vi "Autoarrange Plots.vi"(0 "Data in":T7, 5 "Display State":T3, 9 "panel":refnum<vi>) -> (4 "Data out":T2(array[cluster]), 15 "error out":errorcluster)   [LabVIEW 2015, in "Interactive Graph.xctl"]
uses:
  Interactive Graph.xctl
  Data.vi
  EPhys/LV Source/Work Panel VIs/Typedefs/EPhysWork-Label Position.ctl
  State.vi
  Persistent.ctl
  Plot.ctl
  Events.ctl
  Selection.ctl
  XRange.ctl
  YScale.ctl
  Cursor.ctl
  <vilib>/Analysis/baseanly.llb/Mean (DBL).vi
  <vilib>/Analysis/NI_AALBase.lvlib
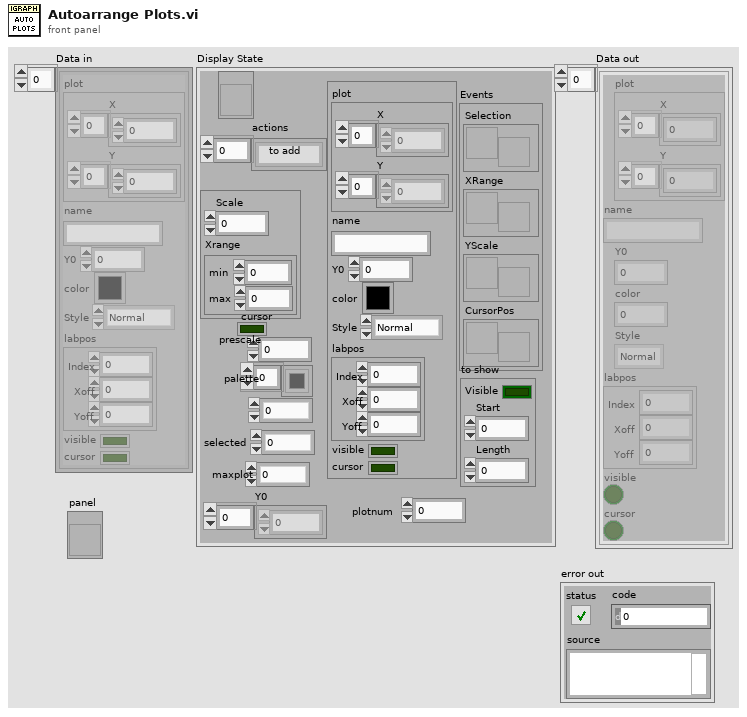
[diagram p1: front panel]
types:
  T1 = typedef "EPhysWork-Label Position.ctl" = cluster{"Index":i32, "Xoff":dbl, "Yoff":dbl}
  T2 = cluster{"plot":cluster{"X":dbl[], "Y":dbl[]}, "name":string, "Y0":dbl, "color":u32, "Style":enum16{"Normal", "Highlight", "Shadow"}, "labpos":T1, "visible":bool, "cursor":bool}[]
  T3 = typedef "Interactive Graph.xctl/State.vi" = cluster{"ref":refnum<vi>, "actions":string[], "Persist":T4, "cursor":bool, "prescale":dbl, "palette":u32[], "colIndex":i32, "to add":T5, "Events":T6, "selected":i32, "to show":cluster{"Visible":bool, "Start":i32, "Length":i32}, "maxplot":i32, "Y0":dbl[], "plotnum":i32}
  T4 = typedef "Interactive Graph.xctl/Persistent.ctl" = cluster{"Scale":dbl, "Xrange":cluster{"min":dbl, "max":dbl}}
  T5 = typedef "Interactive Graph.xctl/Plot.ctl" = cluster{"plot":cluster{"X":dbl[], "Y":dbl[]}, "name":string, "Y0":dbl, "color":u32, "Style":enum16{"Normal", "Highlight", "Shadow"}, "labpos":T1, "visible":bool, "cursor":bool}
  T6 = typedef "Interactive Graph.xctl/Events.ctl" = cluster{"Selection":refnum<user-event>, "XRange":refnum<user-event>, "YScale":refnum<user-event>, "CursorPos":refnum<user-event>}
  T7 = typedef "Interactive Graph.xctl/Data.vi" = cluster{"plot":cluster{"X":dbl[], "Y":dbl[]}, "name":string, "Y0":dbl, "color":u32, "Style":enum16{"Normal", "Highlight", "Shadow"}, "labpos":T1, "visible":bool, "cursor":bool}[]
  T8 = cluster{"plot":cluster{"X":dbl[], "Y":dbl[]}, "name":string, "Y0":dbl, "color":u32, "Style":enum16{"Normal", "Highlight", "Shadow"}, "labpos":T1, "visible":bool, "cursor":bool}
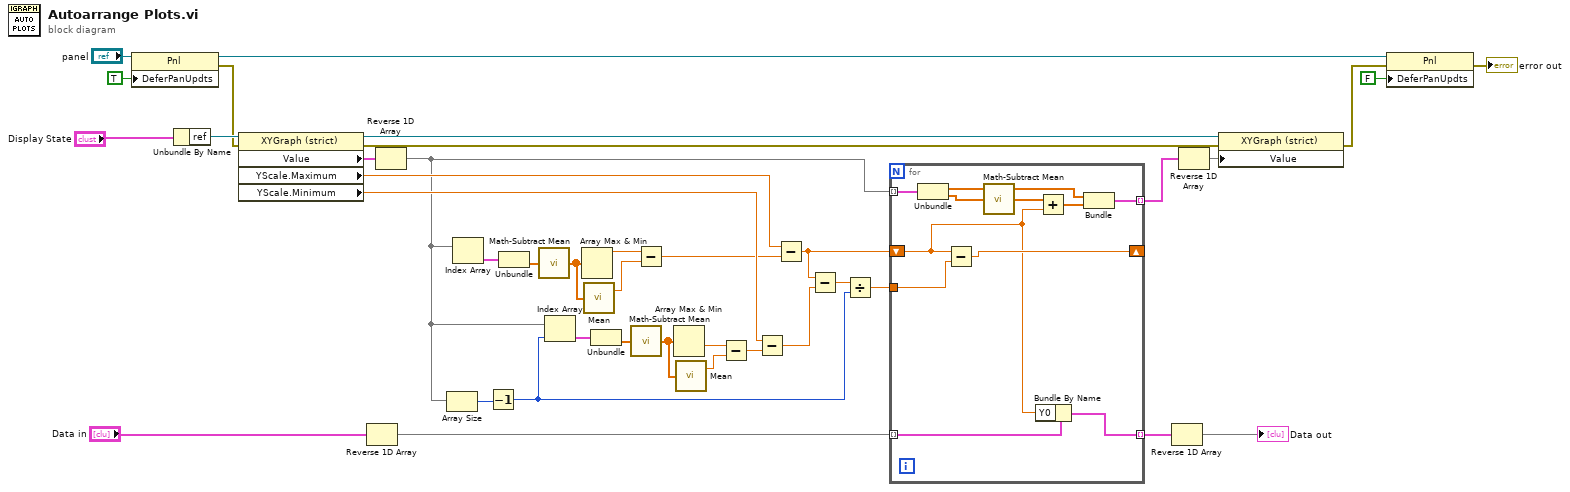
[diagram p0: block diagram]
diagram:
  n1 = property class="Pnl"(reference="panel", "DeferPanUpdts"=TRUE ("Defer Panel Updates")) -> (reference out=w36:refnum<vi>, error out=w7:errorcluster)  [unwired: 1 in]
  n2 = Unbundle By Name("Display State") -> ("ref"=w9:refnum<vi>)
  n3 = property class="XYGraph (strict)"(reference=w9, error in=w7) -> (reference out=w27:refnum<vi>, error out=w28:errorcluster, "Value"=w29:cluster{dbl[], dbl[]}[], "YScale.Maximum"=w30:dbl, "YScale.Minimum"=w31:dbl)
  n4 = Reverse 1D Array(array="Data in") -> (reversed array=w3:T7)
  n5 = Reverse 1D Array(array=w29) -> (reversed array=w4:cluster{dbl[], dbl[]}[])
  n6 = Array Size(array=w4) -> (size(s)=w26:i32)
  n7 = Index Array(array=w4) -> (element=w24:cluster{dbl[], dbl[]})  [unwired: 1 in]
  n8 = Decrement(x=w26) -> (x-1=w32:i32)
  n9 = Unbundle(w24) -> (w23:dbl[])  [unwired: 1 out]
  n10 = call "Math-Subtract Mean.vi"("Y"=w23) -> ("Y - mean(Y)"=w22:dbl[])  [unwired: 4 in]
  n11 = Index Array(array=w4, index=w32) -> (element=w19:cluster{dbl[], dbl[]})
  n12 = Array Max & Min(array=w22) -> (max value=w21:dbl)  [unwired: 3 out]
  n13 = call-poly <vilib>:"Mean.vi"("X"=w22) -> ("mean"=w20:dbl)  [unwired: 1 out]
  n14 = Unbundle(w19) -> (w18:dbl[])  [unwired: 1 out]
  n15 = call "Math-Subtract Mean.vi"("Y"=w18) -> ("Y - mean(Y)"=w17:dbl[])  [unwired: 4 in]
  n16 = Subtract(x=w21, y=w20) -> (x-y=w25:dbl)
  n17 = Array Max & Min(array=w17) -> (min value=w15:dbl)  [unwired: 3 out]
  n18 = call-poly <vilib>:"Mean.vi"("X"=w17) -> ("mean"=w16:dbl)  [unwired: 1 out]
  n19 = Subtract(x=w15, y=w16) -> (x-y=w14:dbl)
  n20 = Subtract(x=w31, y=w14) -> (x-y=w12:dbl)
  n21 = Subtract(x=w30, y=w25) -> (x-y=w13:dbl)
  n22 = Subtract(x=w13, y=w12) -> (x-y=w11:dbl)
  n23 = Divide(x=w11, y=w32) -> (x/y=w10:dbl)
  n24 = for {
    shift-right: [w50] -> _
    shift-left: w13 -> [w41]
    tunnel: w10 -> [w49]
    tunnel: w4 -> [w44] mode=indexing
    tunnel: [w43] -> w33 mode=indexing
    tunnel: w3 -> [w42] mode=indexing
    tunnel: [w40] -> w5 mode=indexing
    n25 = Unbundle(w44) -> (w46:dbl[], w48:dbl[])
    n26 = Subtract(x=w41, y=w49) -> (x-y=w50:dbl)
    n27 = call "Math-Subtract Mean.vi"("Y"=w48) -> ("Y - mean(Y)"=w45:dbl[])  [unwired: 4 in]
    n28 = Bundle By Name(cluster=w42, "Y0"=w41) -> (w40:T8)
    n29 = Add(x=w45, y=w41) -> (x+y=w47:dbl[])
    n30 = Bundle(w46, w47) -> (w43:cluster{dbl[], dbl[]})  [unwired: 1 in]
  }
  n31 = Reverse 1D Array(array=w5) -> (reversed array=→"Data out":T2)
  n32 = Reverse 1D Array(array=w33) -> (reversed array=w1:cluster{dbl[], dbl[]}[])
  n33 = property class="XYGraph (strict)"(reference=w27, error in=w28, "Value"=w1) -> (error out=w8:errorcluster)  [unwired: 1 out]
  n34 = property class="Pnl"(reference=w36, error in=w8, "DeferPanUpdts"=FALSE ("Defer Panel Updates")) -> (error out=→"error out":errorcluster)  [unwired: 1 out]
